vi "Error_manager.vi"(8 "error in (no error)":errorcluster, 10 "Caller VI":refnum<vi>, 11 "Dali_usb_tridonics in":refnum<class "Dali_usb_tridonics.lvclass">) -> (0 "error out":errorcluster, 1 "source":string, 2 "code":i32, 3 "Dali_usb_tridonics out":refnum<class "Dali_usb_tridonics.lvclass">, 5 "Step":string)   [LabVIEW 2014, in "Driver_interaction.lvlib" / "Dali_usb_tridonics.lvclass"]
uses:
  Dali_usb_tridonics.lvclass
  _Driver_interaction/_Driver_interaction.lvclass/_Driver_interaction.ctl
  _Driver_interaction/_Driver_interaction.lvclass
  Deploy/Utilities/Miscelanous.lvlibp
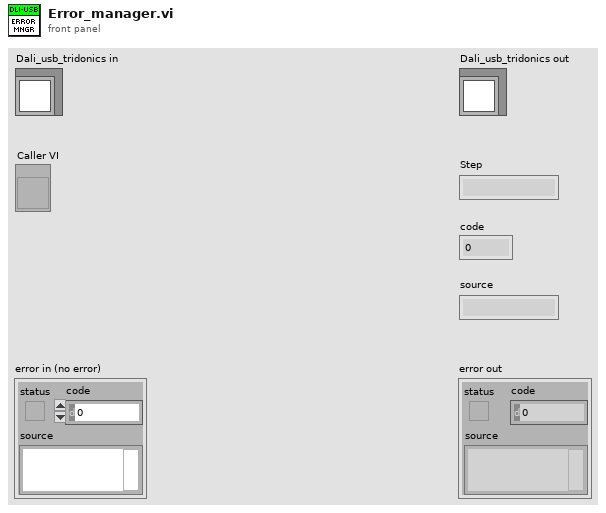
[diagram p1: front panel]
types:
  T1 = typedef "Driver_interaction.lvlib/_Driver_interaction.lvclass/Interface_type.ctl" = string
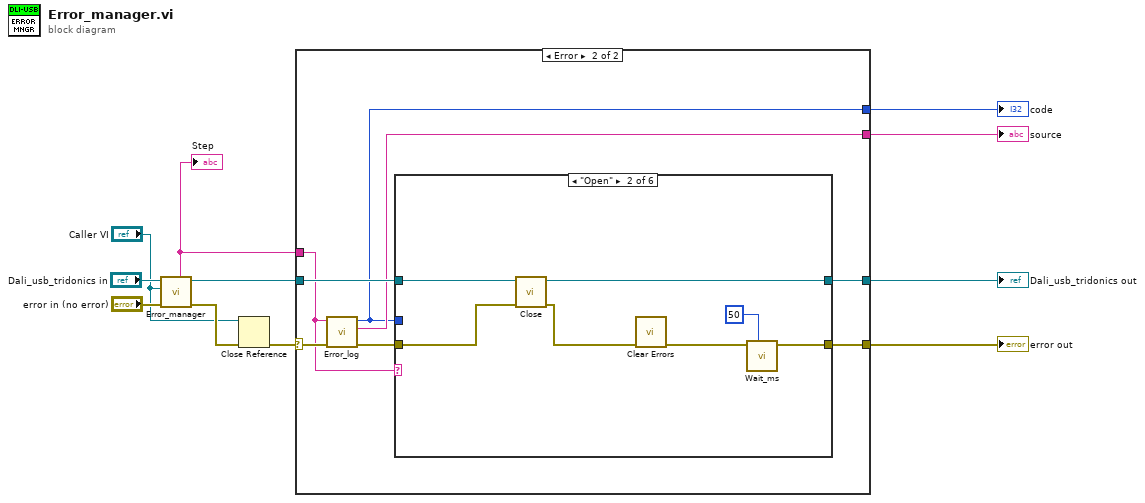
[diagram p0: block diagram]
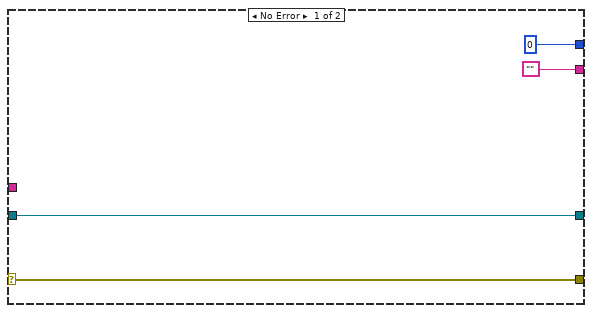
[diagram p2: hidden frame]
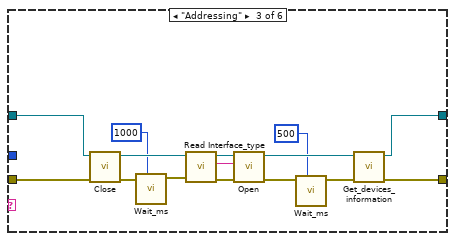
[diagram p4: hidden frame]
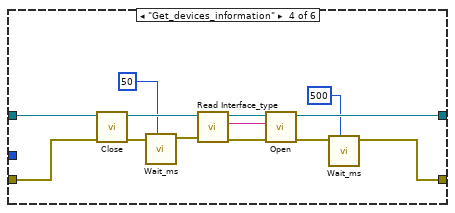
[diagram p5: hidden frame]
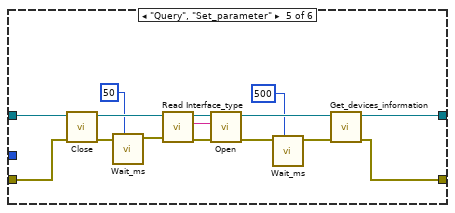
[diagram p6: hidden frame]
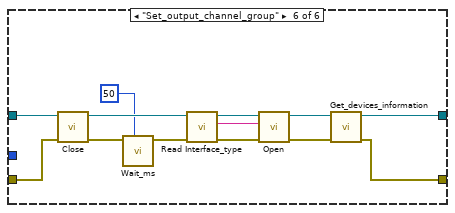
[diagram p7: hidden frame]
diagram:
  n1 = call-parent "Error_manager.vi"("error in (no error)"="error in (no error)", "Caller VI"="Caller VI", "_Driver_interaction in"="Dali_usb_tridonics in") -> ("error out"=w8:errorcluster, "_Driver_interaction out"=w5:refnum<class "Dali_usb_tridonics.lvclass">, "Step"=w4:string)  [unwired: 4 in, 2 out]
  "Step" <- w4
  n2 = Close Reference(reference="Caller VI", error in (no error)=w8) -> (error out=w9:errorcluster)
  n3 = case shown="Error" w9 {
    selector: w9 -> [w15 w23]
    tunnel: w4 -> [_ w16]
    tunnel: w5 -> [w14 w21]
    tunnel: [w14 w20] -> w6
    tunnel: [w15 w19] -> w7
    tunnel: [0 ("code") w17] -> w3
    tunnel: ["" w18] -> w2
    frame No Error {
    }
    frame Error {
      n4 = call "Error_log.vi"("error in (no error)"=w23, "Step"=w16) -> ("error out"=w22:errorcluster, "source"=w18:string, "code"=w17:i32)  [unwired: 7 in]
      n5 = case shown="\"Open\"" w16 {
        tunnel: w22 -> [w28 w35 w41 w65 w74 w86]
        tunnel: w17 -> [w27 _ _ _ _ _]
        tunnel: w21 -> [w26 w37 w39 w64 w80 w93]
        tunnel: [w25 w36 w38 w63 w72 w84] -> w20
        tunnel: [w24 w33 w40 w56 w73 w85] -> w19
        frame Default {
          # "If the issue is triggered in \"Step_name\" method"
          n6 = case shown="Default" w27 {
            tunnel: w28 -> [w29]
            tunnel: w26 -> [w30]
            tunnel: [w30] -> w25
            tunnel: [w29] -> w24
            frame Default {
              # "Create specific solutions to error code"
            }
          }
        }
        frame "Open" {
          n7 = call-dynamic "Close.vi"("error in (no error)"=w35, "Dali_usb_tridonics in"=w37) -> ("error out"=w34:errorcluster, "Dali_usb_tridonics out"=w36:refnum<class "Dali_usb_tridonics.lvclass">)  [unwired: 8 in]
          n8 = call <vilib>:"Clear Errors.vi"("error in (no error)"=w34) -> ("error out"=w31:errorcluster)  [unwired: 5 in, 1 out]
          n9 = call "Wait_ms.vi"("ms to wait"=u32 50, "error in (no error)"=w31) -> ("error out"=w33:errorcluster)  [unwired: 9 in]
        }
        frame "Addressing" {
          n10 = call-dynamic "Close.vi"("error in (no error)"=w41, "Dali_usb_tridonics in"=w39) -> ("error out"=w44:errorcluster, "Dali_usb_tridonics out"=w52:refnum<class "Dali_usb_tridonics.lvclass">)  [unwired: 8 in]
          n11 = call "Wait_ms.vi"("ms to wait"=u32 1000, "error in (no error)"=w44) -> ("error out"=w43:errorcluster)  [unwired: 9 in]
          n12 = call "Read Interface_type.vi"("error in (no error)"=w43, "_Driver_interaction in"=w52) -> ("error out"=w49:errorcluster, "Interface_type"=w48:T1, "_Driver_interaction out"=w51:refnum<class "Dali_usb_tridonics.lvclass">)  [unwired: 7 in]
          n13 = call-dynamic "Open.vi"("error in (no error)"=w49, "Interface_type"=w48, "Dali_usb_tridonics in"=w51) -> ("error out"=w47:errorcluster, "Dali_usb_tridonics out"=w50:refnum<class "Dali_usb_tridonics.lvclass">)  [unwired: 7 in]
          n14 = call "Wait_ms.vi"("ms to wait"=u32 500, "error in (no error)"=w47) -> ("error out"=w46:errorcluster)  [unwired: 9 in]
          n15 = call-dynamic "Get_devices_information.vi"("error in (no error)"=w46, "Dali_usb_tridonics in"=w50) -> ("error out"=w40:errorcluster, "Dali_usb_tridonics out"=w38:refnum<class "Dali_usb_tridonics.lvclass">)  [unwired: 7 in, 1 out]
        }
        frame "Get_devices_information" {
          n16 = call-dynamic "Close.vi"("error in (no error)"=w65, "Dali_usb_tridonics in"=w64) -> ("error out"=w55:errorcluster, "Dali_usb_tridonics out"=w62:refnum<class "Dali_usb_tridonics.lvclass">)  [unwired: 8 in]
          n17 = call "Wait_ms.vi"("ms to wait"=u32 50, "error in (no error)"=w55) -> ("error out"=w54:errorcluster)  [unwired: 9 in]
          n18 = call "Read Interface_type.vi"("error in (no error)"=w54, "_Driver_interaction in"=w62) -> ("error out"=w59:errorcluster, "Interface_type"=w60:T1, "_Driver_interaction out"=w61:refnum<class "Dali_usb_tridonics.lvclass">)  [unwired: 7 in]
          n19 = call-dynamic "Open.vi"("error in (no error)"=w59, "Interface_type"=w60, "Dali_usb_tridonics in"=w61) -> ("error out"=w57:errorcluster, "Dali_usb_tridonics out"=w63:refnum<class "Dali_usb_tridonics.lvclass">)  [unwired: 7 in]
          n20 = call "Wait_ms.vi"("ms to wait"=u32 500, "error in (no error)"=w57) -> ("error out"=w56:errorcluster)  [unwired: 9 in]
        }
        frame "Query", "Set_parameter" {
          n21 = call-dynamic "Close.vi"("error in (no error)"=w74, "Dali_usb_tridonics in"=w80) -> ("error out"=w68:errorcluster, "Dali_usb_tridonics out"=w79:refnum<class "Dali_usb_tridonics.lvclass">)  [unwired: 8 in]
          n22 = call "Wait_ms.vi"("ms to wait"=u32 50, "error in (no error)"=w68) -> ("error out"=w67:errorcluster)  [unwired: 9 in]
          n23 = call "Read Interface_type.vi"("error in (no error)"=w67, "_Driver_interaction in"=w79) -> ("error out"=w76:errorcluster, "Interface_type"=w75:T1, "_Driver_interaction out"=w78:refnum<class "Dali_usb_tridonics.lvclass">)  [unwired: 7 in]
          n24 = call-dynamic "Open.vi"("error in (no error)"=w76, "Interface_type"=w75, "Dali_usb_tridonics in"=w78) -> ("error out"=w71:errorcluster, "Dali_usb_tridonics out"=w77:refnum<class "Dali_usb_tridonics.lvclass">)  [unwired: 7 in]
          n25 = call "Wait_ms.vi"("ms to wait"=u32 500, "error in (no error)"=w71) -> ("error out"=w70:errorcluster)  [unwired: 9 in]
          n26 = call-dynamic "Get_devices_information.vi"("error in (no error)"=w70, "Dali_usb_tridonics in"=w77) -> ("error out"=w73:errorcluster, "Dali_usb_tridonics out"=w72:refnum<class "Dali_usb_tridonics.lvclass">)  [unwired: 7 in, 1 out]
        }
        frame "Set_output_channel_group" {
          n27 = call-dynamic "Close.vi"("error in (no error)"=w86, "Dali_usb_tridonics in"=w93) -> ("error out"=w82:errorcluster, "Dali_usb_tridonics out"=w92:refnum<class "Dali_usb_tridonics.lvclass">)  [unwired: 8 in]
          n28 = call "Wait_ms.vi"("ms to wait"=u32 50, "error in (no error)"=w82) -> ("error out"=w83:errorcluster)  [unwired: 9 in]
          n29 = call "Read Interface_type.vi"("error in (no error)"=w83, "_Driver_interaction in"=w92) -> ("error out"=w88:errorcluster, "Interface_type"=w87:T1, "_Driver_interaction out"=w91:refnum<class "Dali_usb_tridonics.lvclass">)  [unwired: 7 in]
          n30 = call-dynamic "Open.vi"("error in (no error)"=w88, "Interface_type"=w87, "Dali_usb_tridonics in"=w91) -> ("error out"=w89:errorcluster, "Dali_usb_tridonics out"=w90:refnum<class "Dali_usb_tridonics.lvclass">)  [unwired: 7 in]
          n31 = call-dynamic "Get_devices_information.vi"("error in (no error)"=w89, "Dali_usb_tridonics in"=w90) -> ("error out"=w85:errorcluster, "Dali_usb_tridonics out"=w84:refnum<class "Dali_usb_tridonics.lvclass">)  [unwired: 7 in, 1 out]
        }
      }
    }
  }
  "error out" <- w7
  "Dali_usb_tridonics out" <- w6
  "code" <- w3
  "source" <- w2
